vi "Get Step Index.vi"(8 "error in (no error)":errorcluster, 11 "Tester in":refnum<class "Tester.lvclass">) -> (0 "error out":errorcluster, 2 "Step Index":i32, 3 "Tester out":refnum<class "Tester.lvclass">)   [LabVIEW 2020, in "Tester.lvlib" / "Tester.lvclass"]
uses:
  Tester.lvclass
  Tester.lvclass/Tester.ctl
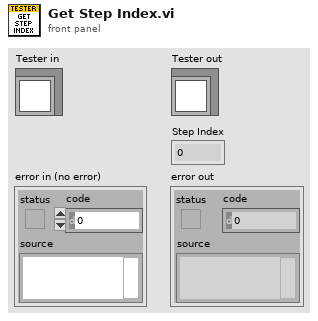
[diagram p1: front panel]
types:
  T1 = typedef "Tester.lvlib/Tester.lvclass/Execution Ref.ctl" = cluster{"Sequence":refnum<class "Sequence.lvclass">, "Step":i32, "Results":refnum<class "Results.lvclass">, "State":T2, "Run Step VI":refnum<vi>, "Abort":bool}
  T2 = typedef "Tester.lvlib/Tester.lvclass/State.ctl" = enum16{"Idle", "In Progress", "Completed"}
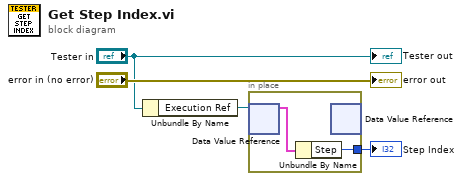
[diagram p0: block diagram]
diagram:
  n1 = Unbundle By Name("Tester in") -> ("Execution Ref"=w3:refnum<data-value>)
  n2 = in-place {
    in-place-border: [w5] -> w1
    n3 = in-place-dvr #1(w3) -> (w6:T1)  [unwired: 1 out]
    n4 = Unbundle By Name(w6) -> ("Step"=w5:i32)
    n5 = in-place-dvr #1() -> ()  [unwired: 1 in, 2 out]
  }
  "Step Index" <- w1
  "error out" <- "error in (no error)"
  "Tester out" <- "Tester in"
